vi "Read Bool.vi"(8 "Error In":errorcluster, 11 "Reader In":refnum<class "Reader.lvclass">) -> (0 "Error Out":errorcluster, 2 "Value":bool, 3 "Reader Out":refnum<class "Reader.lvclass">)   [LabVIEW 2019, in "LabPack.lvlib" / "Reader.lvclass"]
doc: "Reads and decodes a boolean from the MessagePack data."
uses:
  Reader.lvclass
  Reader.lvclass/Reader.ctl
  Status/Read Status.vi
  Status/Read Status Message.vi
  Status/Read Is Error.vi
  Utility/Status Code.vi
  <vilib>/Utility/error.llb/Error Cluster From Error Code.vi
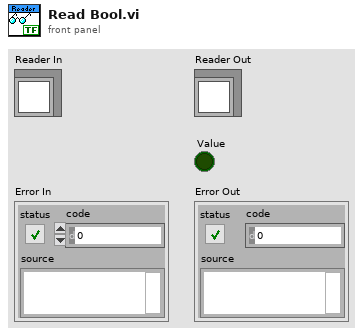
[diagram p1: front panel]
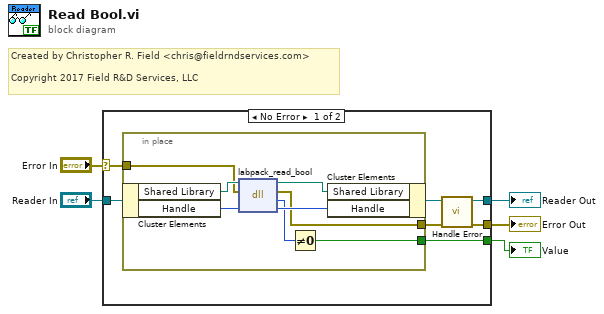
[diagram p0: block diagram]
diagram:
  # "Created by Christopher R. Field <chris@fieldrndservices.com>\n\nCopyright 2017 Field R&D Services, LLC"
  n1 = case shown="No Error" "Error In" {
    selector: "Error In" -> [w11 w21]
    tunnel: "Reader In" -> [w12 w22]
    tunnel: [w7 w21] -> w3
    tunnel: [w9 w22] -> w2
    tunnel: [w6 _] -> w1
    frame No Error {
      n2 = in-place {
        in-place-border: w11 -> [w16]
        in-place-border: [w15] -> w8
        in-place-border: [w13] -> w6
        n3 = in-place-cluster #1(w12) -> ("Shared Library"=w20:path, "Handle"=w18:u64)
        n4 = dll-call lib="D:/Users/cfield/Code/MessagePack/LabPack/LabVIEW/trunk/src/LabPack/Private/labpack-x64.dll" fn="labpack_read_bool"(path in=w20, error in=w16, "reader"=w18) -> (path out=w19:path, error out=w15:errorcluster, "return type"=w14:i32, "reader"=w17:u64)  [unwired: 1 in]
        n5 = Not Equal To 0?(x=w14) -> (x != 0?=w13:bool)
        n6 = in-place-cluster #1("Shared Library"=w19, "Handle"=w17) -> (w10:refnum<class "Reader.lvclass">)
      }
      n7 = call "Handle Error.vi"("Error In"=w8, "Reader In"=w10) -> ("Error Out"=w7:errorcluster, "Reader Out"=w9:refnum<class "Reader.lvclass">)  [unwired: 8 in]
    }
    frame Error {
    }
  }
  "Error Out" <- w3
  "Reader Out" <- w2
  "Value" <- w1
